vi "Open Customized Ini Tokens Folder.vi"   [LabVIEW 2012, in "NEVSTOP_QuickDrop.lvlib"]
uses:
  NEVSTOP_QuickDrop.lvlib
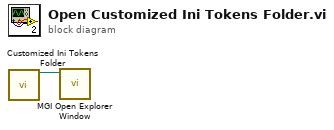
[diagram p0: block diagram]
diagram:
  n1 = call "Customized Ini Tokens Folder.vi"() -> ("appended path"=w1:path)  [unwired: 19 in]
  n2 = call <userlib>:"MGI Open Explorer Window.vi"("Directory or File"=w1) -> ()  [unwired: 10 in, 1 out]
